vi "CheckForCpp2013Redist.vi"(8 "error in (no error)":errorcluster) -> (0 "error out":errorcluster, 2 "Installed":bool)   [LabVIEW 2019]
uses:
  <vilib>/registry/registry.llb/Registry SAM.ctl
  <vilib>/registry/registry.llb/Registry RtKey.ctl
  <vilib>/registry/registry.llb/Read Registry Value Simple U32.vi
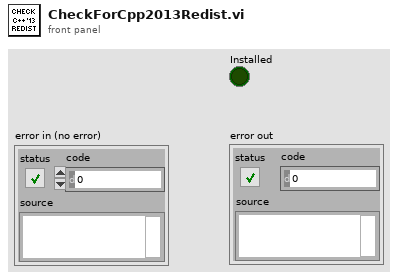
[diagram p1: front panel]
types:
  T1 = typedef "Registry RtKey.ctl" = enum32{"HKEY_CLASSES_ROOT", "HKEY_CURRENT_USER", "HKEY_LOCAL_MACHINE", "HKEY_USERS", "HKEY_PERFORMANCE_DATA", "HKEY_CURRENT_CONFIG", "HKEY_DYN_DATA"}
  T2 = typedef "Registry SAM.ctl" = enum32{"KEY_QUERY_VALUE", "KEY_SET_VALUE", "KEY_CREATE_SUB_KEY", "KEY_ENUMERATE_SUB_KEYS", "KEY_NOTIFY", "KEY_CREATE_LINK", "KEY_READ", "KEY_WRITE", "KEY_ALL_ACCESS", "KEY_READ | KEY_WRITE"}
  T3 = typedef "Registry refnum.ctl" = refnum<k1>
  T4 = cluster{"numSubKeys":i32, "maxSubKeyLen":i32, "maxSubKeyClassLen":i32}
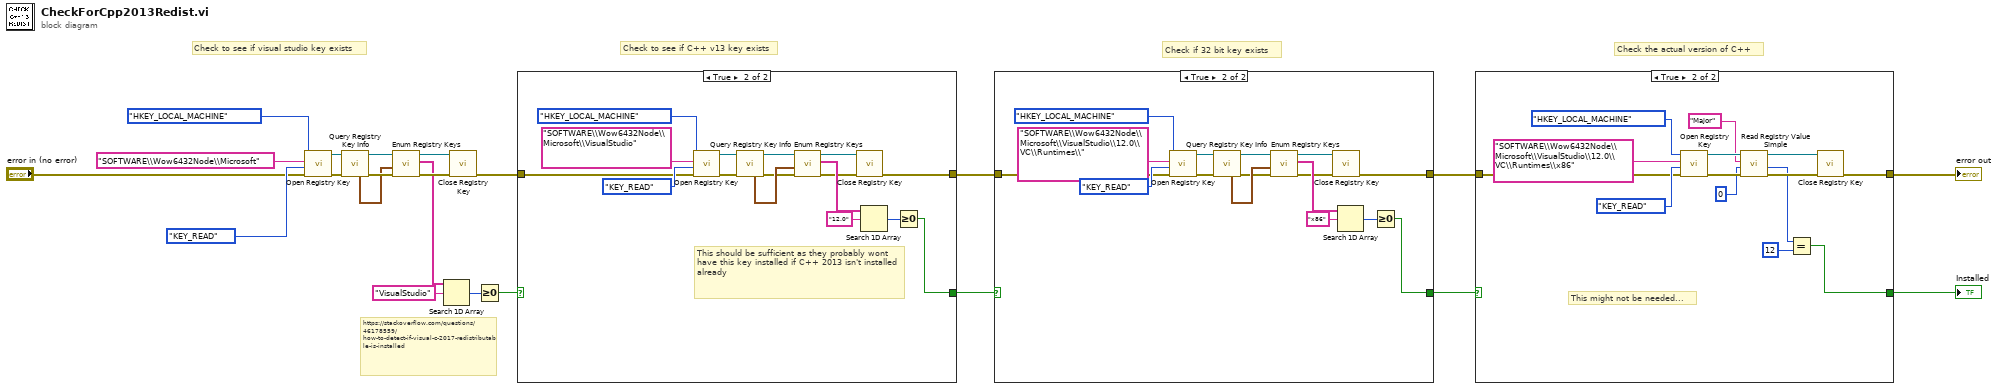
[diagram p0: block diagram]
diagram:
  # "Check if 32 bit key exists"
  # "Check the actual version of C++"
  # "Check to see if C++ v13 key exists"
  # "Check to see if visual studio key exists"
  # "https://stackoverflow.com/questions/46178559/how-to-detect-if-visual-c-2017-redistributable-is-installed"
  n1 = call <vilib>:"Open Registry Key.vi"("error in (no error)"="error in (no error)", "security access mask (KEY_READ | KEY_WRITE)"=Registry_SAM."KEY_READ", "subkey"="SOFTWARE\\Wow6432Node\\Microsoft", "root key (HKEY_LOCAL_MACHINE)"=Registry_RtKey."HKEY_LOCAL_MACHINE") -> ("error out"=w21:errorcluster, "refnum out"=w22:T3)  [unwired: 6 in]
  n2 = call <vilib>:"Query Registry Key Info.vi"("error in (no error)"=w21, "refnum"=w22) -> ("error out"=w19:errorcluster, "refnum out"=w20:T3, "subkey info"=w13:T4)  [unwired: 5 in, 2 out]
  n3 = call <vilib>:"Enum Registry Keys.vi"("error in (no error)"=w19, "subkey info"=w13, "refnum"=w20) -> ("error out"=w17:errorcluster, "subkeys"=w12:string[], "refnum out"=w18:T3)  [unwired: 6 in]
  n4 = Search 1D Array(1D array=w12, element="VisualStudio") -> (index of element=w10:i32)  [unwired: 1 in]
  n5 = call <vilib>:"Close Registry Key.vi"("error in (no error)"=w17, "refnum"=w18) -> ("error out"=w9:errorcluster)  [unwired: 5 in]
  n6 = Greater Or Equal To 0?(x=w10) -> (x >= 0?=w8:bool)
  n7 = case shown="True" w8 {
    selector: w8 -> [w24 _]
    tunnel: w9 -> [w23 w27]
    tunnel: [w24 w25] -> w5
    tunnel: [w23 w26] -> w4
    frame False {
    }
    frame True {
      # "This should be sufficient as they probably wont have this key installed if C++ 2013 isn't installed already"
      n8 = call <vilib>:"Open Registry Key.vi"("error in (no error)"=w27, "security access mask (KEY_READ | KEY_WRITE)"=Registry_SAM."KEY_READ", "subkey"="SOFTWARE\\Wow6432Node\\Microsoft\\VisualStudio", "root key (HKEY_LOCAL_MACHINE)"=Registry_RtKey."HKEY_LOCAL_MACHINE") -> ("error out"=w29:errorcluster, "refnum out"=w28:T3)  [unwired: 6 in]
      n9 = call <vilib>:"Query Registry Key Info.vi"("error in (no error)"=w29, "refnum"=w28) -> ("error out"=w31:errorcluster, "refnum out"=w30:T3, "subkey info"=w37:T4)  [unwired: 5 in, 2 out]
      n10 = call <vilib>:"Enum Registry Keys.vi"("error in (no error)"=w31, "subkey info"=w37, "refnum"=w30) -> ("error out"=w33:errorcluster, "subkeys"=w38:string[], "refnum out"=w32:T3)  [unwired: 6 in]
      n11 = call <vilib>:"Close Registry Key.vi"("error in (no error)"=w33, "refnum"=w32) -> ("error out"=w26:errorcluster)  [unwired: 5 in]
      n12 = Search 1D Array(1D array=w38, element="12.0") -> (index of element=w40:i32)  [unwired: 1 in]
      n13 = Greater Or Equal To 0?(x=w40) -> (x >= 0?=w25:bool)
    }
  }
  n14 = case shown="True" w5 {
    selector: w5 -> [w42 _]
    tunnel: w4 -> [w41 w45]
    tunnel: [w42 w43] -> w2
    tunnel: [w41 w44] -> w3
    frame False {
    }
    frame True {
      n15 = call <vilib>:"Open Registry Key.vi"("error in (no error)"=w45, "security access mask (KEY_READ | KEY_WRITE)"=Registry_SAM."KEY_READ", "subkey"="SOFTWARE\\Wow6432Node\\Microsoft\\VisualStudio\\12.0\\VC\\Runtimes\\", "root key (HKEY_LOCAL_MACHINE)"=Registry_RtKey."HKEY_LOCAL_MACHINE") -> ("error out"=w47:errorcluster, "refnum out"=w46:T3)  [unwired: 6 in]
      n16 = call <vilib>:"Query Registry Key Info.vi"("error in (no error)"=w47, "refnum"=w46) -> ("error out"=w49:errorcluster, "refnum out"=w48:T3, "subkey info"=w55:T4)  [unwired: 5 in, 2 out]
      n17 = call <vilib>:"Enum Registry Keys.vi"("error in (no error)"=w49, "subkey info"=w55, "refnum"=w48) -> ("error out"=w51:errorcluster, "subkeys"=w56:string[], "refnum out"=w50:T3)  [unwired: 6 in]
      n18 = call <vilib>:"Close Registry Key.vi"("error in (no error)"=w51, "refnum"=w50) -> ("error out"=w44:errorcluster)  [unwired: 5 in]
      n19 = Search 1D Array(1D array=w56, element="x86") -> (index of element=w58:i32)  [unwired: 1 in]
      n20 = Greater Or Equal To 0?(x=w58) -> (x >= 0?=w43:bool)
    }
  }
  n21 = case shown="True" w2 {
    selector: w2 -> [w60 _]
    tunnel: w3 -> [w59 w66]
    tunnel: [w60 w61] -> w7
    tunnel: [w59 w65] -> w6
    frame False {
    }
    frame True {
      # "This might not be needed..."
      n22 = call <vilib>:"Open Registry Key.vi"("error in (no error)"=w66, "security access mask (KEY_READ | KEY_WRITE)"=Registry_SAM."KEY_READ" ("security access mask"), "subkey"="SOFTWARE\\Wow6432Node\\Microsoft\\VisualStudio\\12.0\\VC\\Runtimes\\x86", "root key (HKEY_LOCAL_MACHINE)"=Registry_RtKey."HKEY_LOCAL_MACHINE") -> ("error out"=w74:errorcluster, "refnum out"=w72:T3)  [unwired: 6 in]
      n23 = call-poly <vilib>:"Read Registry Value Simple.vi"("error in (no error)"=w74, "default data"=u32 0, "value"="Major", "refnum"=w72) -> ("error out"=w73:errorcluster, "DWORD data"=w64:u32, "refnum out"=w71:T3)  [unwired: 2 in, 1 out]
      n24 = Equal?(x=w64, y=u32 12) -> (x = y?=w61:bool)
      n25 = call <vilib>:"Close Registry Key.vi"("error in (no error)"=w73, "refnum"=w71) -> ("error out"=w65:errorcluster)  [unwired: 5 in]
    }
  }
  "Installed" <- w7
  "error out" <- w6
